vi "Read Value (variant).vi"(8 "error in (no error)":errorcluster, 11 "U32 D Element in":refnum<class "U32 D Element.lvclass">) -> (0 "error out":errorcluster, 2 "Variant":variant, 3 "U32 D Element out":refnum<class "U32 D Element.lvclass">)   [LabVIEW 2018, in "D Datagrid Library.lvlib" / "U32 D Element.lvclass"]
uses:
  U32 D Element.lvclass
  U32 D Element.lvclass/U32 D Element.ctl
  Read Value.vi
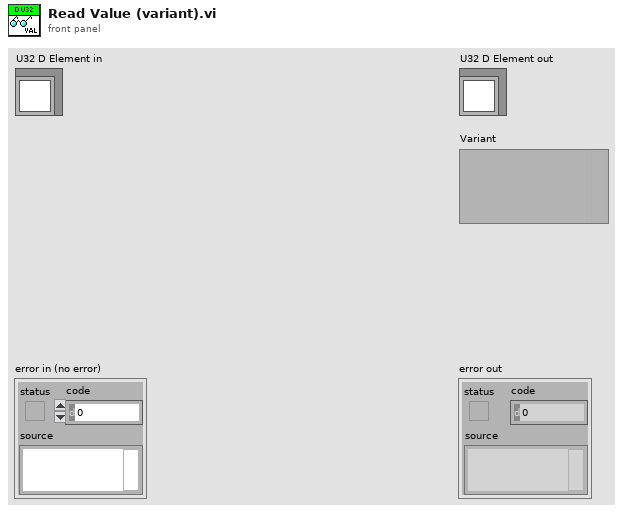
[diagram p1: front panel]
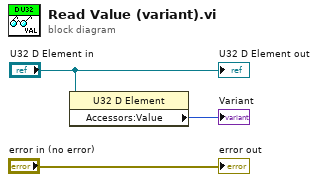
[diagram p0: block diagram]
diagram:
  n1 = property class="U32 D Element"(reference="U32 D Element in") -> ("Accessors:Value"=→"Variant":u32)  [unwired: 1 in, 2 out]
  "error out" <- "error in (no error)"
  "U32 D Element out" <- "U32 D Element in"
